vi "Test_MemoryCtrl.vi"() -> ()   [LabVIEW 2020]
panel:
  out "init data value":dbl=42.0
  out "new data value":dbl
  out "data value reference":refnum<data-value>
  out "free memory":u64
  out "total memory":u64
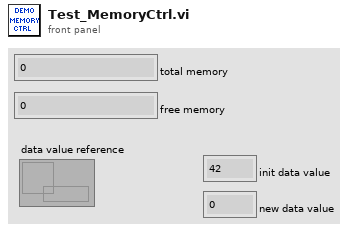
[diagram p1: front panel]
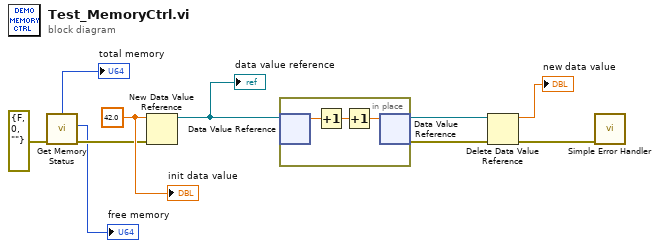
[diagram p0: block diagram]
diagram:
  w10 = 42.0 ("data value")
  n1 = call <vilib>:"Get Memory Status.vi"("error in (no error)"=errorcluster {"status"=FALSE, "code"=0, "source"=""}) -> ("error out"=w8:errorcluster, "free physical memory"=→"free memory":u64, "total physical memory"=→"total memory":u64)  [unwired: 7 in, 1 out]
  n2 = New Data Value Reference(data value=w10, error in=w8) -> (data value reference=w5:refnum<data-value>)  [unwired: 1 out]
  "data value reference" <- w5
  n3 = in-place {
    n4 = in-place-dvr #1(w5) -> (w13:dbl)  [unwired: 1 out]
    n5 = Increment(x=w13) -> (x+1=w12:dbl)
    n6 = Increment(x=w12) -> (x+1=w11:dbl)
    n7 = in-place-dvr #1(w11) -> (w4:refnum<data-value>, w3:errorcluster)
  }
  n8 = Delete Data Value Reference(data value reference=w4, error in=w3) -> (data value=→"new data value":dbl, error out=w1:errorcluster)
  n9 = call <vilib>:"Simple Error Handler.vi"("error in (no error)"=w1) -> ()  [unwired: 4 in, 5 out]
  "init data value" <- w10
